vi "SwissSPAD Live_Get Detector PCB Version.vi"(8 "error in (no error)":errorcluster, 11 "serialNumber":string) -> (0 "error out":errorcluster, 1 "Sensor Part":string, 2 "PCB Version":T1, 3 "serialNumber (dup)":string)   [LabVIEW 2021]
doc: "Reads FPGA Database.txt to figure out which code to send to the firmware based on the <B>Bitfile Type</B> field associated with each FPGA <B>S/N</B>"
uses:
  SwissSPAD Live_SSx PCB Version.ctl
  <vilib>/Utility/error.llb/Error Cluster From Error Code.vi
  <vilib>/ErrorRing/Error Ring.xnode
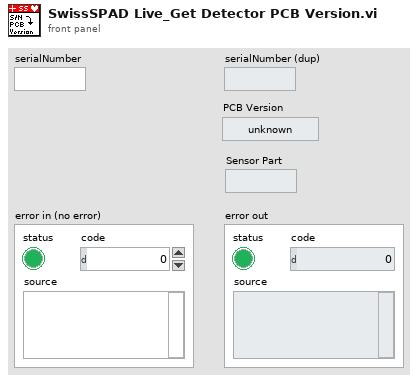
[diagram p1: front panel]
types:
  T1 = typedef "SwissSPAD Live_SSx PCB Version.ctl" = enum16{"unknown", "SS2 PCB1", "SS2 PCB2", "SS3 PCB1"}
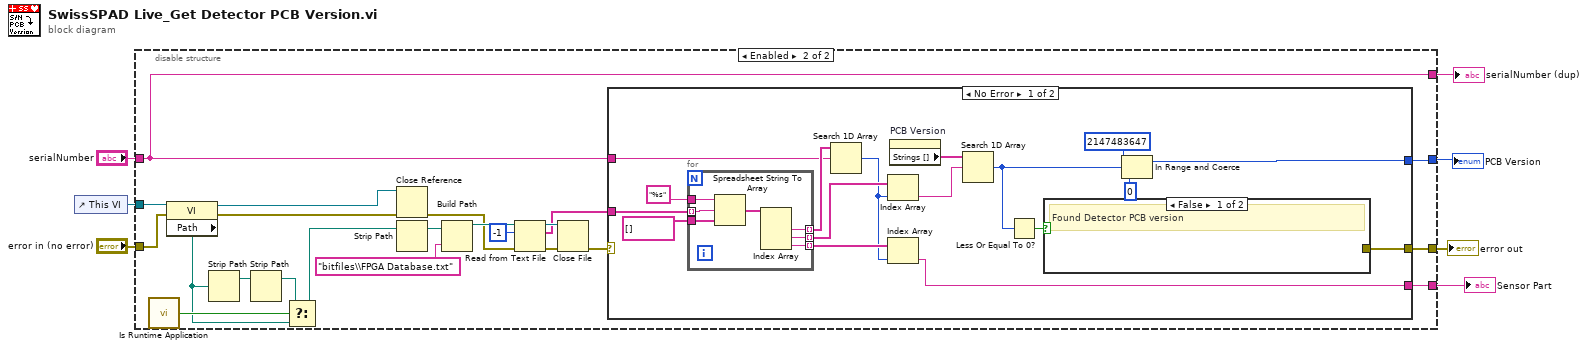
[diagram p0: block diagram]
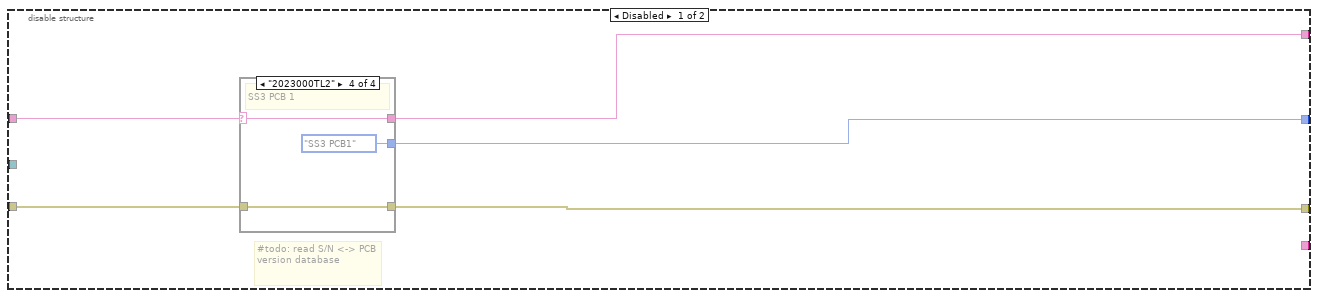
[diagram p2: hidden frame]
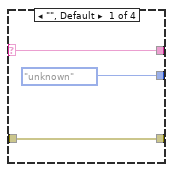
[diagram p3: hidden frame]
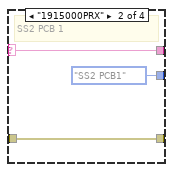
[diagram p4: hidden frame]
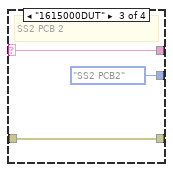
[diagram p5: hidden frame]
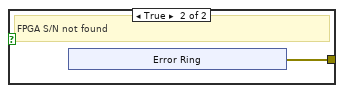
[diagram p6: hidden frame]
diagram:
  n1 = control-ref of="This VI"() -> (w2:refnum<vi>)
  n2 = disable-structure shown="Enabled" {
    disable-tunnel: "error in (no error)" -> [w12 w45]
    disable-tunnel: [w11 w31] -> w6
    disable-tunnel: "serialNumber" -> [w10 w34]
    disable-tunnel: [w9 w34] -> w4
    disable-tunnel: [w8 w33] -> w3
    disable-tunnel: w2 -> [_ w46]
    disable-tunnel: [_ w25] -> w1
    frame Disabled {
      # "#todo: read S/N <-> PCB version database"
      n3 = case shown="\"2023000TL2\"" w10 {
        selector: w10 -> [w15 w16 w19 w22]
        tunnel: [w13 w18 w21 w24] -> w11
        tunnel: [w15 w16 w19 w22] -> w9
        tunnel: [SwissSPAD_Live_SSx_PCB_Version."unknown" ("PCB Version") SwissSPAD_Live_SSx_PCB_Version."SS2 PCB1" ("PCB Version") SwissSPAD_Live_SSx_PCB_Version."SS2 PCB2" ("PCB Version") SwissSPAD_Live_SSx_PCB_Version."SS3 PCB1" ("PCB Version")] -> w8
        tunnel: w12 -> [w13 w18 w21 w24]
        frame "", Default {
        }
        frame "1915000PRX" {
          # "SS2 PCB 1"
        }
        frame "1615000DUT" {
          # "SS2 PCB 2"
        }
        frame "2023000TL2" {
          # "SS3 PCB 1"
        }
      }
    }
    frame Enabled {
      n4 = call "Is Runtime Application.vi"() -> ("Runtime ?"=w28:bool)  [unwired: 8 in, 1 out]
      n5 = property class="VI"(reference=w46, error in=w45) -> (reference out=w39:refnum<vi>, error out=w41:errorcluster, "Path"=w27:path)
      n6 = Strip Path(path=w27) -> (stripped path=w30:path)  [unwired: 1 out]
      n7 = Strip Path(path=w30) -> (stripped path=w29:path)  [unwired: 1 out]
      n8 = Select(t=w29, s=w28, f=w27) -> (s? t:f=w26:path)
      n9 = Close Reference(reference=w39, error in (no error)=w41) -> (error out=w40:errorcluster)
      n10 = Strip Path(path=w26) -> (stripped path=w44:path)  [unwired: 1 out]
      n11 = Build Path(base path=w44, name or relative path="bitfiles\\FPGA Database.txt") -> (appended path=w42:path)
      n12 = Read from Text File(file (use dialog)=w42, count=-1, error in=w40) -> (refnum out=w36:refnum<file>, text=w35:string[], error out=w38:errorcluster)  [unwired: 1 in, 1 out]
      n13 = Close File(refnum=w36, error in=w38) -> (error out=w32:errorcluster)  [unwired: 1 out]
      n14 = case shown="No Error" w32 {
        selector: w32 -> [_ w76]
        tunnel: w35 -> [w62 _]
        tunnel: w34 -> [w60 _]
        tunnel: [w52 _] -> w33
        tunnel: [w54 w76] -> w31
        tunnel: [w47 _] -> w25
        frame No Error {
          n15 = for {
            tunnel: w62 -> [w75] mode=indexing
            tunnel: "%s" ("format string") -> [w74]
            tunnel: string[] [] ("text") -> [w72]
            tunnel: [w71] -> w61 mode=indexing
            tunnel: [w70] -> w59 mode=indexing
            tunnel: [w69] -> w49 mode=indexing
            n16 = Spreadsheet String To Array(format string=w74, spreadsheet string=w75, array type (2D Dbl)=w72) -> (array=w73:string[])  [unwired: 1 in]
            n17 = Index Array(array=w73) -> (element #1=w71:string, element #2=w70:string, element #3=w69:string)  [unwired: 3 in]
          }
          n18 = Search 1D Array(1D array=w61, element=w60) -> (index of element=w48:i32)  [unwired: 1 in]
          n19 = Index Array(array=w59, index=w48) -> (element=w57:string)
          n20 = Index Array(array=w49, index=w48) -> (element=w47:string)
          n21 = property on="PCB Version" class="Enum (strict)"() -> ("Strings []"=w58:string[])  [unwired: 2 in, 2 out]
          n22 = Search 1D Array(1D array=w58, element=w57) -> (index of element=w56:i32)  [unwired: 1 in]
          n23 = Less Or Equal To 0?(x=w56) -> (x <= 0?=w55:bool)
          n24 = case shown="False" w55 {
            tunnel: [_ w64] -> w54
            frame False {
              # "Found Detector PCB version"
            }
            frame True {
              # "FPGA S/N not found"
              n25 = xnode "Error Ring"() -> ("error out"=w64:errorcluster)
            }
          }
          n26 = In Range and Coerce(upper limit=2147483647, x=w56, lower limit=0) -> (coerced(x)=w52:i32)  [unwired: 1 out]
        }
        frame Error {
          # "FPGA Database not found"
        }
      }
    }
  }
  "PCB Version" <- w3
  "serialNumber (dup)" <- w4
  "error out" <- w6
  "Sensor Part" <- w1
